vi "Open Current VI Location.vi"(6 "Variant in":variant, 7 "Shift Pressed?":bool, 8 "error in (no error)":errorcluster, 10 "QD Combo Box Ref":refnum<vi>, 11 "QD Launch VI Ref":refnum<vi>) -> (0 "error out":errorcluster, 4 "Variant out":variant)   [LabVIEW 2014, in "NEVSTOP_QuickDrop.lvlib"]
doc: "Open Current VI Location in Explorer Window."
uses:
  NEVSTOP_QuickDrop.lvlib
  <userlib>/_OpenG.lib/file/file.llb/Valid Path - Traditional__ogtk.vi
panel:
  in  "Undo Name":string="NEVSTOP__OpenFileLocaiton"
  # "Do not change the connector pane of this VI.\n\nSee the block diagram for directions on how to use this template."
  # "Specify the name of the Undo transaction"
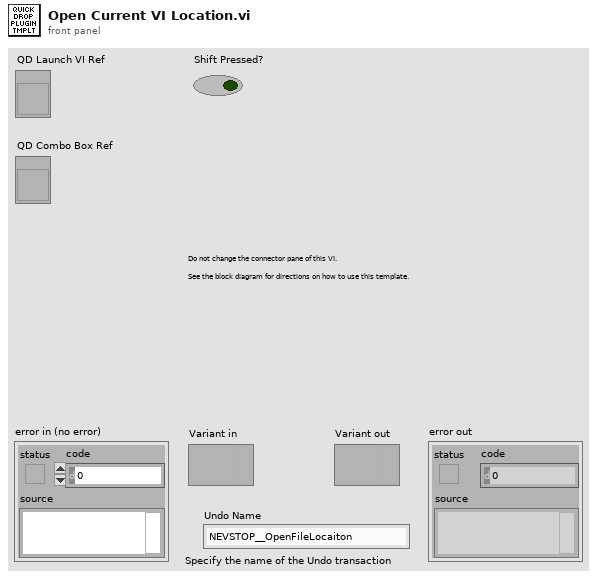
[diagram p1: front panel]
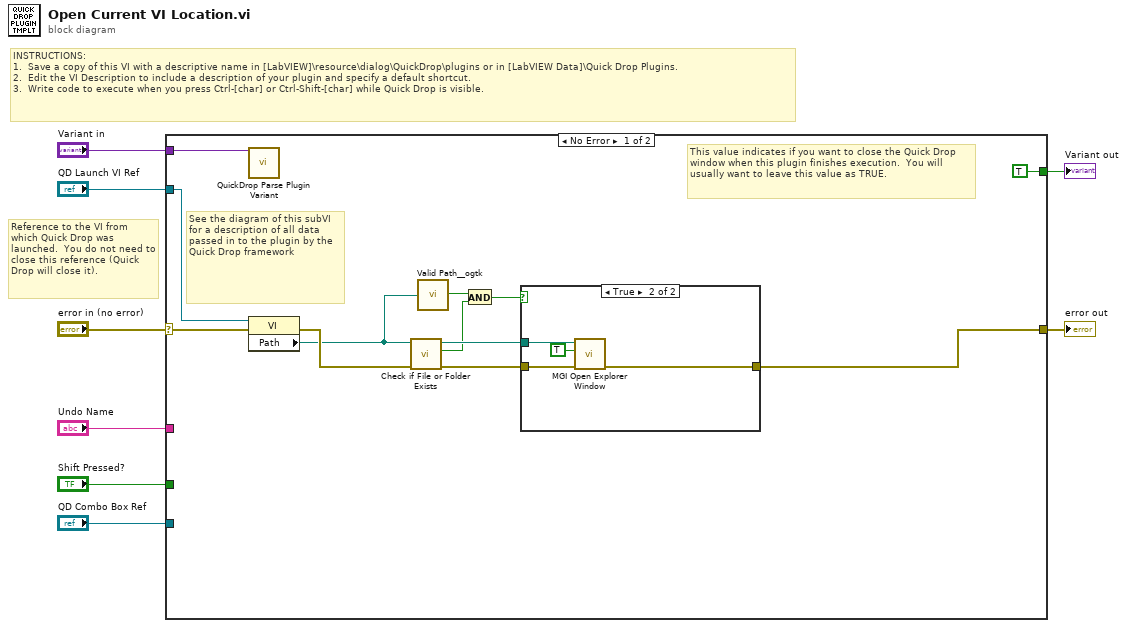
[diagram p0: block diagram]
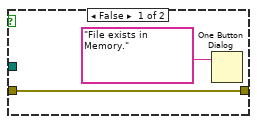
[diagram p2: hidden frame]
diagram:
  # "Reference to the VI from which Quick Drop was launched.  You do not need to close this reference (Quick Drop will close it)."
  # "INSTRUCTIONS:\n1.  Save a copy of this VI with a descriptive name in [LabVIEW]\\resource\\dialog\\QuickDrop\\plugins or in [LabVIEW Data]\\Quick Drop Plugins.\n2.  Edit the VI Description to include a description of your plugin and specify a default shortcut. \n3.  Write code to execute when you press Ctrl-[char] or Ctrl-Shift-[char] while Quick Drop is visible."
  n1 = case shown="No Error" "error in (no error)" {
    selector: "error in (no error)" -> [w19 w27]
    tunnel: [w16 w27] -> w7
    tunnel: "QD Launch VI Ref" -> [w18 _]
    tunnel: "Shift Pressed?" -> [_ _]
    tunnel: "QD Combo Box Ref" -> [_ _]
    tunnel: "Variant in" -> [w20 _]
    tunnel: "Undo Name" -> [_ _]
    tunnel: [TRUE _] -> w1
    frame No Error {
      # "This value indicates if you want to close the Quick Drop window when this plugin finishes execution.  You will usually want to leave this value as TRUE."
      # "See the diagram of this subVI for a description of all data passed in to the plugin by the Quick Drop framework"
      n2 = call <vilib>:"QuickDrop Parse Plugin Variant.vi"("QDKS Variant in"=w20) -> ()  [unwired: 12 in, 3 out]
      n3 = property class="VI"(reference=w18, error in=w19) -> (error out=w14:errorcluster, "Path"=w10:path)  [unwired: 1 out]
      n4 = call <vilib>:"Check if File or Folder Exists.vi"("error in (no error)"=w14, "path"=w10) -> ("error out"=w13:errorcluster, "file or folder exists?"=w11:bool, "dup path"=w15:path)  [unwired: 7 in]
      n5 = call-poly <userlib>:"Valid Path__ogtk.vi"("path"=w10) -> ("valid"=w12:bool)
      n6 = And(x=w12, y=w11) -> (x .and. y?=w9:bool)
      n7 = case shown="True" w9 {
        tunnel: [w22 w25] -> w16
        tunnel: w15 -> [_ w24]
        tunnel: w13 -> [w22 w23]
        frame False {
          n8 = One Button Dialog(message="File exists in Memory.") -> ()  [unwired: 1 in, 1 out]
        }
        frame True {
          n9 = call <userlib>:"MGI Open Explorer Window.vi"("error in (no error)"=w23, "Select Directory? (F: Open Directory)"=TRUE, "Directory or File"=w24) -> ("error out"=w25:errorcluster)  [unwired: 8 in]
        }
      }
    }
    frame Error {
    }
  }
  "error out" <- w7
  "Variant out" <- w1
